vi "Set System Settings.vi"(11 "SystemStartupSettings":T1) -> ()   [LabVIEW 2016, in "RT Management.lvlib" / "RT Management.lvclass"]
uses:
  RT Management.lvclass
  Controls/SystemSettings.ctl
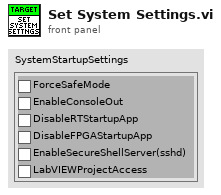
[diagram p1: front panel]
types:
  T1 = typedef "RT Management.lvlib/RT Management.lvclass/SystemSettings.ctl" = cluster{"ForceSafeMode":bool, "EnableConsoleOut":bool, "DisableRTStartupApp":bool, "DisableFPGAStartupApp":bool, "EnableSecureShellServer(sshd)":bool, "LabVIEWProjectAccess":bool}
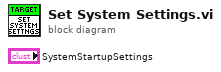
[diagram p0: block diagram]
diagram:
